vi "beep_pc_speaker_lv821.vi"(2 "Duration (seconds)":i32=1000, 3 "Frequency (Hz)":i32=440) -> ()   [LabVIEW 2010]
doc: "Causes the system to issue an audible tone."
uses:
  kernel32.dll
panel:
  # "See block diagram for instructions."
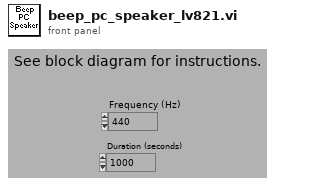
[diagram p1: front panel]
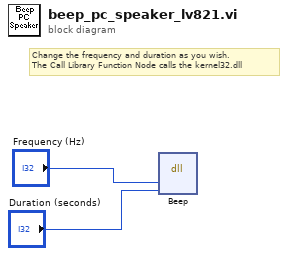
[diagram p0: block diagram]
diagram:
  # "Change the frequency and duration as you wish.\nThe Call Library Function Node calls the kernel32.dll"
  n1 = dll-call lib="KERNEL32.DLL" fn="Beep"("Frequency (Hz)", "Duration (seconds)") -> ()  [unwired: 6 in, 2 out]
